vi "move X.vi"(10 "y mm":dbl, 11 "x mm":dbl) -> (2 "X Position":i32, 3 "Speed X":i32)   [LabVIEW 2016]
uses:
  Settings/Traverse-Settings-Global.vi
  <userlib>/ICNC/ICNC2.lvlib
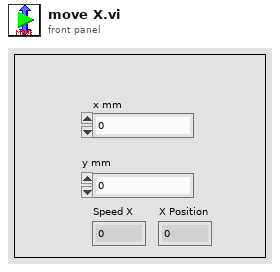
[diagram p1: front panel]
types:
  T1 = cluster{"Acceleration":dbl[], "Deceleration":dbl[], "Max Velocity":dbl[], "Speed":dbl, "Pulse/Degree":dbl, "Degre Factor":dbl[]}
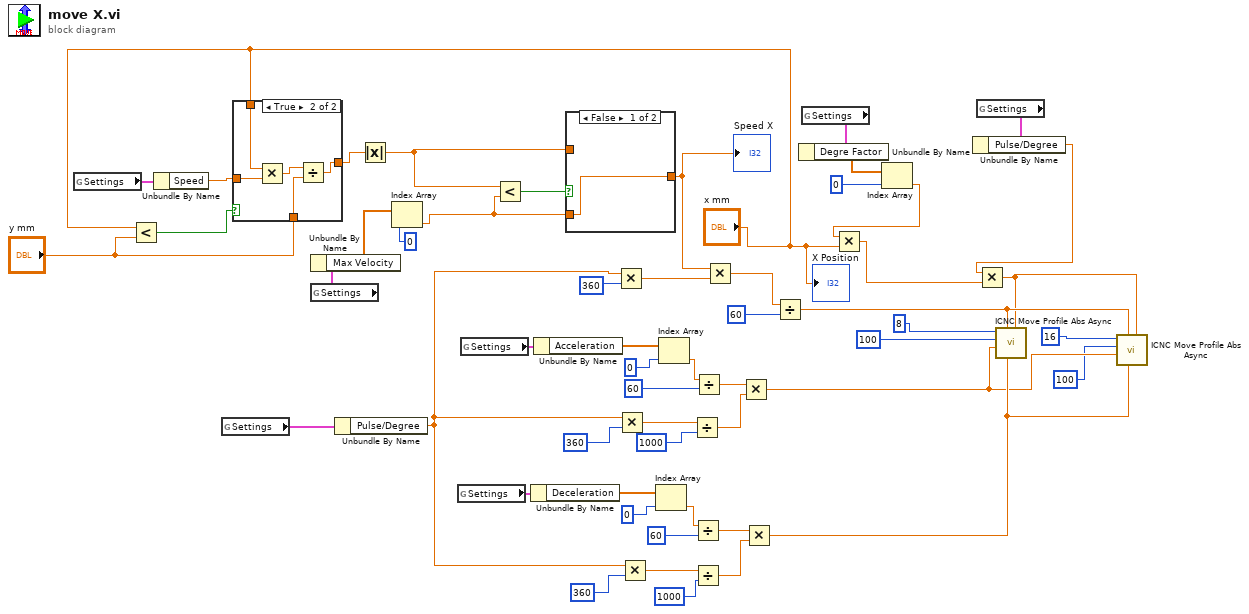
[diagram p0: block diagram]
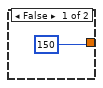
[diagram p2: hidden frame]
diagram:
  n1 = global read "Traverse-Settings-Global.vi" "Settings"() -> (w22:T1)
  n2 = Less?(x="x mm", y="y mm") -> (x < y?=w26:bool)
  n3 = Unbundle By Name(w22) -> ("Speed"=w21:dbl)
  n4 = global read "Traverse-Settings-Global.vi" "Settings"() -> (w20:T1)
  n5 = case shown="True" w26 {
    tunnel: "y mm" -> [_ w57]
    tunnel: [150 w56] -> w25
    tunnel: "x mm" -> [_ w59]
    tunnel: w21 -> [_ w60]
    frame False {
    }
    frame True {
      n6 = Multiply(x=w59, y=w60) -> (x*y=w58:dbl)
      n7 = Divide(x=w58, y=w57) -> (x/y=w56:dbl)
    }
  }
  n8 = global read "Traverse-Settings-Global.vi" "Settings"() -> (w8:T1)
  n9 = Unbundle By Name(w8) -> ("Max Velocity"=w5:dbl[])
  n10 = Unbundle By Name(w20) -> ("Pulse/Degree"=w19:dbl)
  n11 = Absolute Value(x=w25) -> (abs(x)=w24:dbl)
  n12 = Index Array(array=w5, index=0) -> (element=w6:dbl)
  n13 = global read "Traverse-Settings-Global.vi" "Settings"() -> (w14:T1)
  n14 = global read "Traverse-Settings-Global.vi" "Settings"() -> (w18:T1)
  n15 = Less?(x=w24, y=w6) -> (x < y?=w41:bool)
  n16 = Unbundle By Name(w14) -> ("Deceleration"=w13:dbl[])
  n17 = Unbundle By Name(w18) -> ("Acceleration"=w17:dbl[])
  n18 = case shown="False" w41 {
    tunnel: w24 -> [_ w62]
    tunnel: w6 -> [w61 _]
    tunnel: [w61 w62] -> w29
    frame False {
    }
    frame True {
    }
  }
  "Speed X" <- w29
  n19 = Multiply(x=w19, y=360) -> (x*y=w38:dbl)
  n20 = Multiply(x=w19, y=360) -> (x*y=w40:dbl)
  n21 = Multiply(x=w19, y=360) -> (x*y=w39:dbl)
  n22 = Index Array(array=w13, index=0) -> (element=w11:dbl)
  n23 = Index Array(array=w17, index=0) -> (element=w16:dbl)
  n24 = Divide(x=w40, y=1000) -> (x/y=w53:dbl)
  n25 = Divide(x=w11, y=60) -> (x/y=w49:dbl)
  n26 = Divide(x=w39, y=1000) -> (x/y=w48:dbl)
  n27 = Divide(x=w16, y=60) -> (x/y=w43:dbl)
  n28 = Multiply(x=w29, y=w38) -> (x*y=w42:dbl)
  n29 = Multiply(x=w43, y=w53) -> (x*y=w33:dbl)
  n30 = Multiply(x=w49, y=w48) -> (x*y=w34:dbl)
  n31 = Divide(x=w42, y=60) -> (x/y=w35:dbl)
  n32 = global read "Traverse-Settings-Global.vi" "Settings"() -> (w4:T1)
  n33 = Unbundle By Name(w4) -> ("Degre Factor"=w1:dbl[])
  n34 = Index Array(array=w1, index=0) -> (element=w2:dbl)
  n35 = Multiply(x=w2, y="x mm") -> (x*y=w30:dbl)
  n36 = global read "Traverse-Settings-Global.vi" "Settings"() -> (w10:T1)
  n37 = Unbundle By Name(w10) -> ("Pulse/Degree"=w9:dbl)
  n38 = Multiply(x=w9, y=w30) -> (x*y=w28:dbl)
  n39 = call "ICNC Move Profile Abs Async.vi"("Position"=w28, "Decel"=w34, "Speed"=w35, "Accel"=w33, "FStartStop"=100, "Axe"=8) -> ()  [unwired: 4 in, 2 out]
  n40 = call "ICNC Move Profile Abs Async.vi"("Position"=w28, "Decel"=w34, "Speed"=w35, "Accel"=w33, "FStartStop"=100, "Axe"=16) -> ()  [unwired: 4 in, 2 out]
  "X Position" <- "x mm"
